vi "tm_setlut_40.vi"(8 "error in (no error)":errorcluster, 10 "LUT Points":cluster{"In Point":i32, "Out Point":i32}[](array[cluster]), 11 "Handle in":u32) -> (0 "error out":errorcluster, 3 "Handle out":u32)   [LabVIEW 2023]
uses:
  tmcamcon.dll
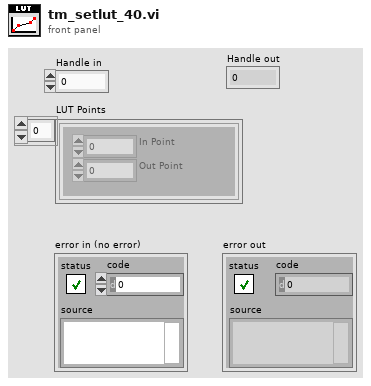
[diagram p1: front panel]
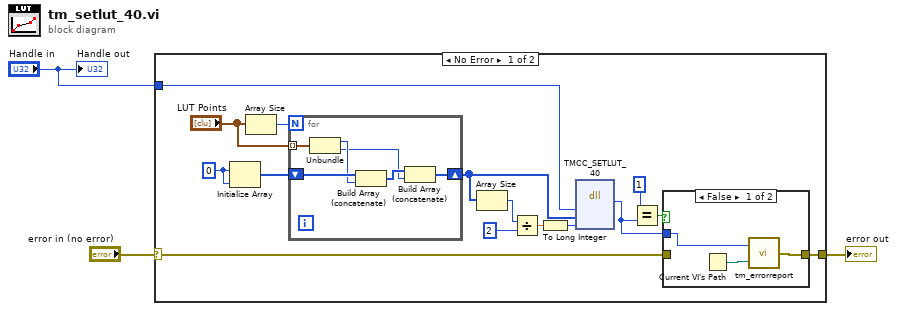
[diagram p0: block diagram]
diagram:
  n1 = case shown="No Error" "error in (no error)" {
    selector: "error in (no error)" -> [w17 w29]
    tunnel: [w16 w29] -> w2
    tunnel: "Handle in" -> [w18 _]
    frame No Error {
      w13 = 0 ("element")
      n2 = Initialize Array(w13, w13) -> (w12:i32[])
      n3 = Array Size(array="LUT Points") -> (size(s)=w15:i32)
      n4 = for {
        N: w15 -> [_]
        tunnel: "LUT Points" -> [w24] mode=indexing
        shift-right: [w19] -> w11
        shift-left: w12 -> [w23]
        n5 = Unbundle(w24) -> ("In Point"=w21:i32, "Out Point"=w20:i32)
        n6 = Build Array (concatenate)(w23, w21) -> (w22:i32[])
        n7 = Build Array (concatenate)(w22, w20) -> (w19:i32[])
      }
      n8 = Array Size(array=w11) -> (size(s)=w10:i32)
      n9 = Divide(x=w10, y=2) -> (x/y=w7:dbl)
      n10 = To Long Integer(number=w7) -> (32bit integer=w8:i32)
      n11 = dll-call lib="tmcamcon.dll" fn="TMCC_SETLUT_40"("HDCAM"=w18, "lutpointarray"=w11, "lutpoints"=w8) -> ("return type"=w5:u32)  [unwired: 6 in, 2 out]
      n12 = Equal?(x=u32 1, y=w5) -> (x = y?=w6:bool)
      n13 = case shown="False" w6 {
        tunnel: w17 -> [_ w28]
        tunnel: [w25 w28] -> w16
        tunnel: w5 -> [w27 _]
        frame False {
          n14 = Current VI's Path() -> (path=w26:path)
          n15 = call "tm_errorreport.vi"("Source"=w26, "Error"=w27) -> ("error out"=w25:errorcluster)
        }
        frame True {
        }
      }
    }
    frame Error {
    }
  }
  "error out" <- w2
  "Handle out" <- "Handle in"
